vi "Export_Data_From_TXT_v1.0.vi"() -> ()   [LabVIEW 2018]
panel:
  out "array":dbl[][](array[numeric])
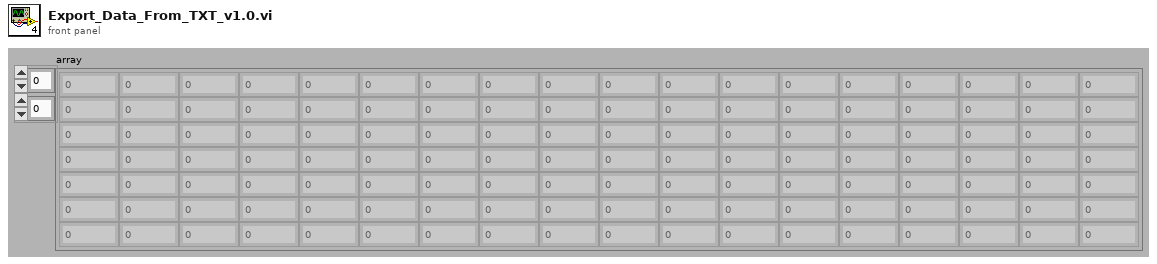
[diagram p1: front panel]
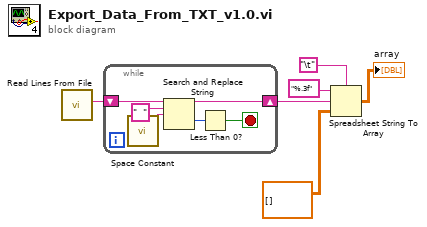
[diagram p0: block diagram]
diagram:
  n1 = call <vilib>:"Read Lines From File.vi"() -> ("line string"=w4:string)  [unwired: 2 in, 7 out]
  n2 = while {
    shift-right: [w9] -> w3
    shift-left: w4 -> [w12]
    stop <- w7 stop-if-true
    n3 = call <vilib>:"Space Constant.vi"() -> ("String"=w10:string)
    n4 = Search and Replace String(input string=w12, search string="  ", replace string=w10) -> (result string=w9:string, offset past replacement=w8:i32)  [unwired: 1 in, 6 out]
    n5 = Less Than 0?(x=w8) -> (x < 0?=w7:bool)
  }
  n6 = Spreadsheet String To Array(delimiter (Tab)="\t", format string="%.3f" ("format (%.3f)"), spreadsheet string=w3, array type (2D Dbl)=dbl[][] [] ("type (empty)")) -> (array=→"array":dbl[][])
